vi "Initialize Data.vi"(8 "Error In":errorcluster, 11 "State In":T1) -> (0 "Error Out":errorcluster, 3 "State Out":T1)   [LabVIEW 2018, in "Bookmark Manager.lvlib"]
uses:
  Bookmark Manager.lvlib
  Controls/State.ctl
  <vilib>/addons/analyzer/_analyzerctrls.llb/VIAnCtl Analysis App Info.ctl
  Controls/Bookmark.ctl
  Controls/VI Identifier.ctl
  Controls/Bookmarks Groups.ctl
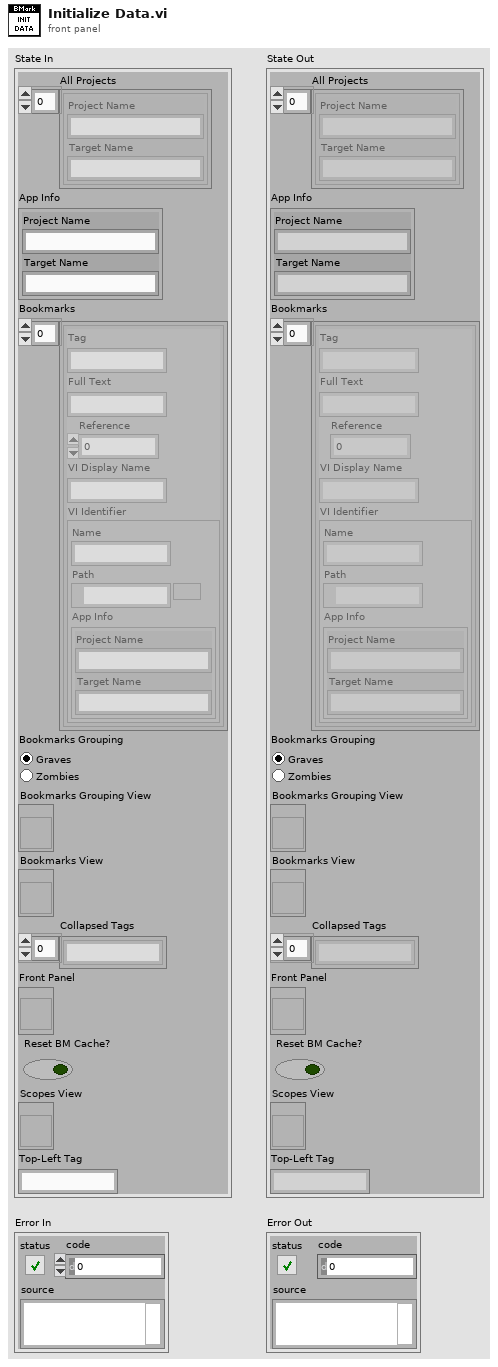
[diagram p1: front panel]
types:
  T1 = typedef "Bookmark Manager.lvlib/State.ctl" = cluster{"All Projects":T2[], "App Info":T2, "Bookmarks":T3[], "Bookmarks Grouping":T5, "Bookmarks Grouping View":refnum<vi>, "Bookmarks View":refnum<vi>, "Collapsed Tags":string[], "Front Panel":refnum<vi>, "Reset BM Cache?":bool, "Scopes View":refnum<vi>, "Top-Left Tag":string}
  T2 = typedef "VIAnCtl Analysis App Info.ctl" = cluster{"Project Name":string, "Target Name":string}
  T3 = typedef "Bookmark Manager.lvlib/Bookmark.ctl" = cluster{"Tag":string, "Full Text":string, "Reference":i32, "VI Display Name":string, "VI Identifier":T4}
  T4 = typedef "Bookmark Manager.lvlib/VI Identifier.ctl" = cluster{"Name":string, "Path":path, "App Info":T2}
  T5 = typedef "Bookmark Manager.lvlib/Bookmarks Groups.ctl" = enum32{"Graves", "Zombies"}
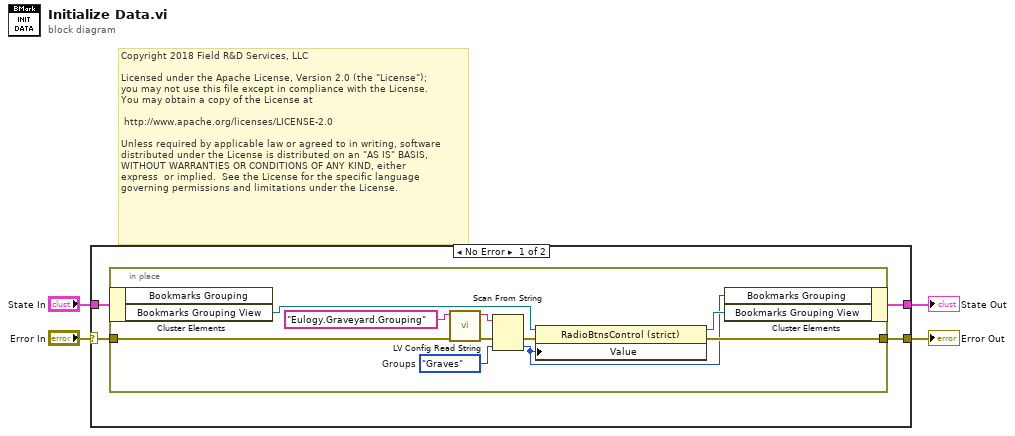
[diagram p0: block diagram]
diagram:
  # "Copyright 2018 Field R&D Services, LLC\n\nLicensed under the Apache License, Version 2.0 (the \"License\");\nyou may not use this file except in compliance with the License.\nYou may obtain a copy of the License at\n\n\thttp://www.apache.org/licenses/LICENSE-2.0\n\nUnless required by applicable law or agreed to in writing, software\ndistributed under the License is distributed on an \"AS IS\" BASIS,\nWITHOUT WARRANTIES OR CONDITIONS OF ANY KIND, either \nexpress  or implied.  See the License for the specific language \ngoverning permissions and limitations under the License."
  n1 = case shown="No Error" "Error In" {
    selector: "Error In" -> [w5 w19]
    tunnel: [w8 w19] -> w4
    tunnel: [w7 w20] -> w3
    tunnel: "State In" -> [w6 w20]
    frame No Error {
      n2 = in-place {
        in-place-border: w5 -> [w14]
        in-place-border: [w16] -> w8
        w11 = Bookmarks_Groups."Graves"  # Groups
        n3 = in-place-cluster #1(w6) -> ("Bookmarks Grouping View"=w18:refnum<vi>)  [unwired: 1 out]
        n4 = call <resource>:"LV Config Read String.vi"("error in"=w14, "key"="Eulogy.Graveyard.Grouping") -> ("error out"=w13:errorcluster, "value"=w10:string)  [unwired: 3 in, 1 out]
        n5 = Scan From String(input string=w10, error in=w13, default 1=w11) -> (error out=w12:errorcluster, output 1=w9:T5)  [unwired: 2 in, 2 out]
        n6 = property class="RadioBtnsControl (strict)"(reference=w18, error in=w12, "Value"=w9) -> (reference out=w17:refnum<vi>, error out=w16:errorcluster)
        n7 = in-place-cluster #1("Bookmarks Grouping"=w9, "Bookmarks Grouping View"=w17) -> (w7:T1)
      }
    }
    frame Error {
    }
  }
  "Error Out" <- w4
  "State Out" <- w3
